vi "pixmap.vi"(8 "Error In":errorcluster, 10 "size":T1, 11 "QIcon In":refnum<class "QIcon.lvclass">) -> (0 "Error Out":errorcluster, 2 "Value":refnum<class "QPixmap.lvclass">, 3 "QIcon Out":refnum<class "QIcon.lvclass">)   [LabVIEW 2014, in "QIcon.lvclass"]
doc: "LabVIEW-specific documentation is not yet available. See <b>http://doc.qt.io/qt-5/QIcon.html#pixmap</b>"
uses:
  QIcon.lvclass
  QPixmap/QPixmap.lvclass
  LQ Core/QSize.ctl
  LQ Core/LQSerialData/LQSerialData.lvclass/LQSerialData.ctl
  LQ Core/LQ Core.lvlib
  LQ Core/LQSerialData/LQSerialData.lvclass
panel:
  # "Copyright (c) 2016 Sze Howe Koh\n\nThis Source Code Form is subject to the terms of the Mozilla Public\nLicense, v. 2.0. If a copy of the MPL was not distributed with this\nfile, You can obtain one at http://mozilla.org/MPL/2.0/."
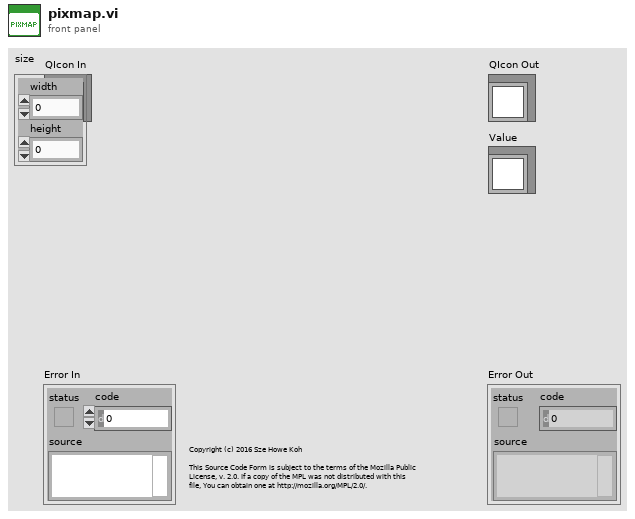
[diagram p1: front panel]
types:
  T1 = typedef "QSize.ctl" = cluster{"width":i32, "height":i32}
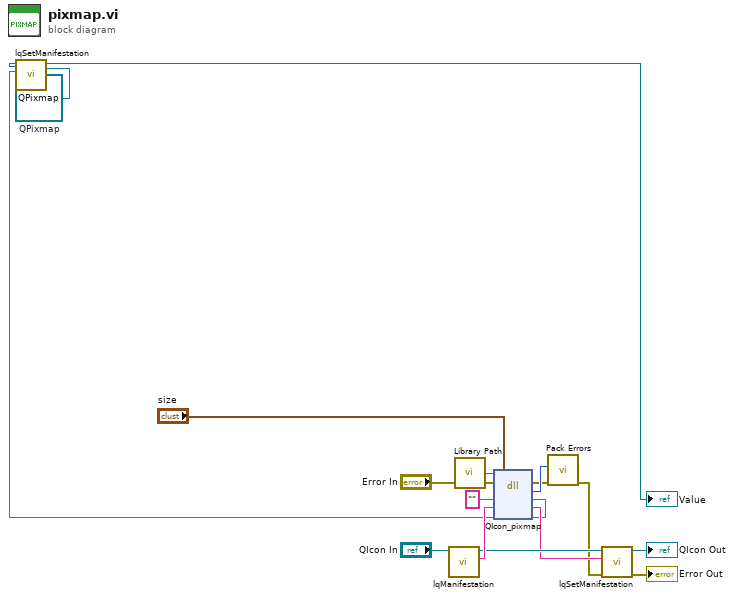
[diagram p0: block diagram]
diagram:
  w2 = refnum<class "QPixmap.lvclass"> refnum  # QPixmap
  n1 = call "lqManifestation.vi"("LQSerialData in"="QIcon In") -> ("Manifestation"=w14:string, "LQSerialData out"=w12:refnum<class "QIcon.lvclass">)  [unwired: 9 in]
  n2 = call "Library Path.vi"() -> ("Library Path"=w9:path)
  n3 = dll-call lib="?" fn="QIcon_pixmap"(path in=w9, error in="Error In", "_retVal"="" ("retVal"), "_instance"=w14, "size"="size") -> (error out=w6:errorcluster, w7:i32, "_retVal"=w3:string, "_instance"=w10:string)  [unwired: 2 in, 1 out]
  n4 = call "lqSetManifestation.vi"("Manifestation"=w3, "LQSerialData in"=w2) -> ("LQSerialData out"=→"Value":refnum<class "QPixmap.lvclass">)  [unwired: 8 in, 1 out]
  n5 = call "Pack Errors.vi"("Error In"=w6, "Error Code"=w7) -> ("Error Out"=w5:errorcluster)  [unwired: 9 in]
  n6 = call "lqSetManifestation.vi"("Error In"=w5, "Manifestation"=w10, "LQSerialData in"=w12) -> ("Error Out"=→"Error Out":errorcluster, "LQSerialData out"=→"QIcon Out":refnum<class "QIcon.lvclass">)  [unwired: 7 in]
